vi "boolean to enable or grayed out.vi"(4 "enable?":bool) -> (1 "state?":T1(ring)=enum."Disabled and Grayed Out")   [LabVIEW 2023, in "Reusable Library.lvlib"]
uses:
  Reusable Library.lvlib
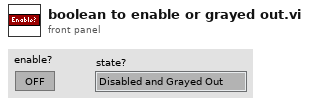
[diagram p1: front panel]
types:
  T1 = enum8{"Enabled", "Disabled", "Disabled and Grayed Out"}
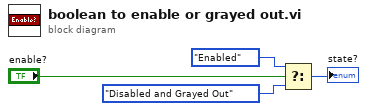
[diagram p0: block diagram]
diagram:
  n1 = Select(t=T1."Enabled" ("Disabled"), s="enable?", f=T1."Disabled and Grayed Out" ("Disabled")) -> (s? t:f=→"state?":T1)
